vi "Unflatten (offset).vi"(8 "error in (no error)":errorcluster, 9 "offset (0)":i32, 10 "JSON stream":string, 11 "JSON Object In":refnum<class "JSON Object.lvclass">) -> (0 "error out":errorcluster, 1 "offset":i32, 3 "JSON Object Out":refnum<class "JSON Object.lvclass">, 4 "Empty?":bool)   [LabVIEW 2011, in "JSON Object.lvclass"]
uses:
  JSON Object.lvclass
  JSON Value/JSON Value.lvclass
  JSON Object.lvclass/JSON Object.ctl
  JSON Scalar/Strip Quotes.vi
  JSON Scalar/Parse In String (offset).vi
  JSON Scalar/Unescape JSON string.vi
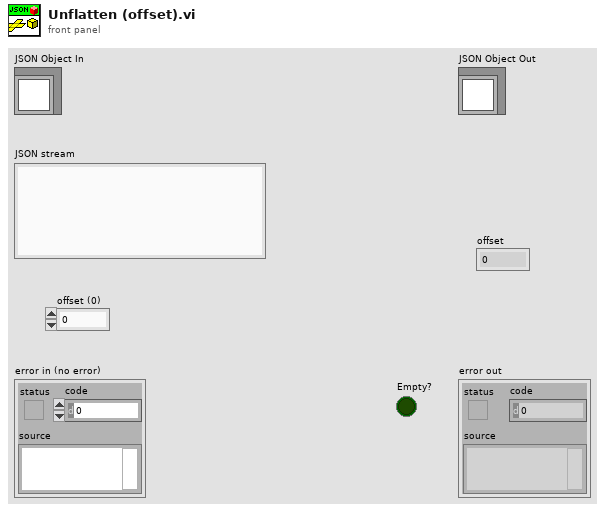
[diagram p1: front panel]
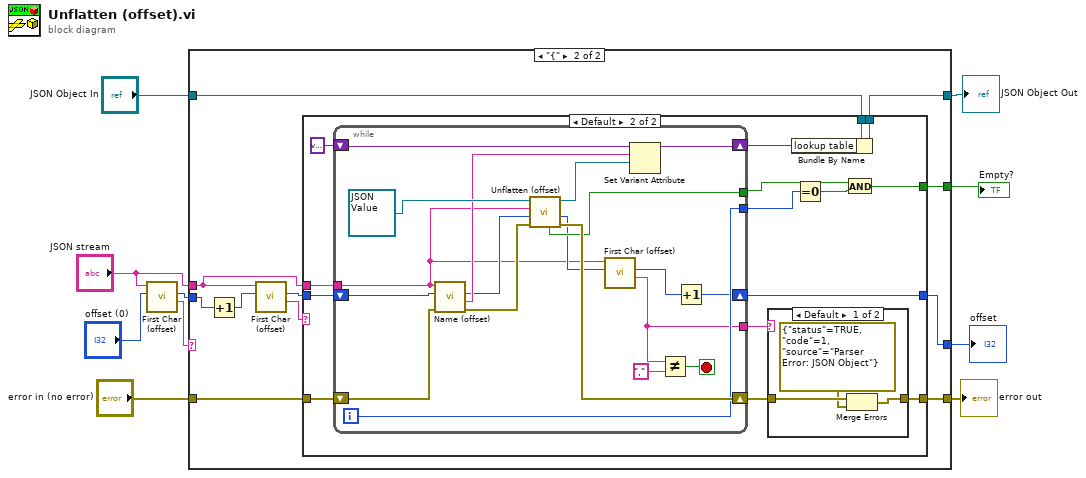
[diagram p0: block diagram]
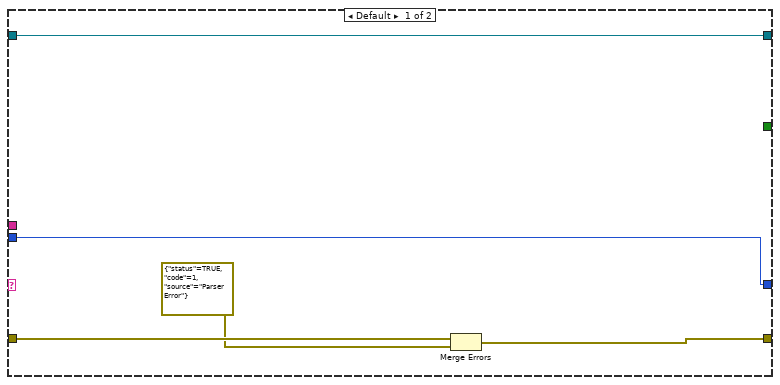
[diagram p2: hidden frame]
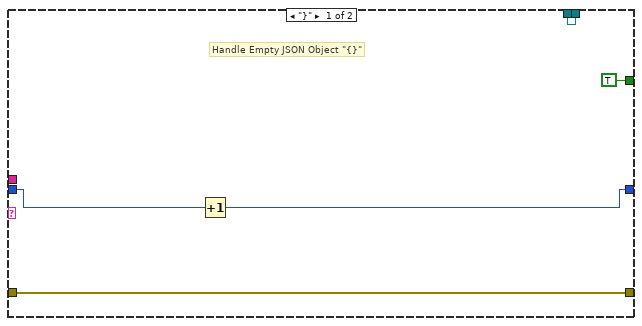
[diagram p3: hidden frame]
diagram:
  n1 = call "First Char (offset).vi"("offset (0)"="offset (0)", "String in"="JSON stream") -> ("First Char"=w10:string, "Offset"=w3:i32)  [unwired: 8 in]
  n2 = case shown="\"{\"" w10 {
    tunnel: "JSON stream" -> [_ w16]
    tunnel: [w15 w23] -> w9
    tunnel: "error in (no error)" -> [w12 w24]
    tunnel: [w14 w25] -> w7
    tunnel: "JSON Object In" -> [w14 w26]
    tunnel: [_ w22] -> w5
    tunnel: w3 -> [w13 w20]
    tunnel: [w13 w17] -> w2
    frame Default {
      n3 = Merge Errors(w12, errorcluster {"status"=TRUE, "code"=1, "source"="Parser Error"} ("error in")) -> (w15:errorcluster)
    }
    frame "{" {
      n4 = Increment(x=w20) -> (x+1=w19:i32)
      n5 = call "First Char (offset).vi"("offset (0)"=w19, "String in"=w16) -> ("First Char"=w21:string, "Offset"=w18:i32)  [unwired: 8 in]
      n6 = case shown="Default" w21 {
        tunnel: w16 -> [_ w46]
        tunnel: w26 -> [w31 w45]
        tunnel: [w31 w44] -> w25
        tunnel: w24 -> [w29 w43]
        tunnel: [w29 w41] -> w23
        tunnel: [TRUE w34] -> w22
        tunnel: w18 -> [w28 w33]
        tunnel: [w27 w32] -> w17
        frame "}" {
          # "Handle Empty JSON Object \"{}\""
          n7 = Increment(x=w28) -> (x+1=w27:i32)
        }
        frame Default {
          n8 = while {
            tunnel: [w58] -> w42
            shift-right: [w67] -> w40
            shift-left: w43 -> [w60]
            shift-right: [w63] -> w38
            shift-left: variant -> [w62]
            tunnel: [w55] -> w36
            tunnel: [w61] -> w37
            shift-right: [w53] -> w32
            shift-left: w33 -> [w57]
            tunnel: w46 -> [w51]
            i -> [w61]
            stop <- w68 stop-if-true
            n9 = call "Name (offset).vi"("error in (no error)"=w60, "offset (0)"=w57, "JSON"=w51) -> ("error out"=w59:errorcluster, "JSON name"=w65:string, "offset"=w56:i32)  [unwired: 6 in]
            n10 = call-dynamic "Unflatten (offset).vi"("error in (no error)"=w59, "offset (0)"=w56, "JSON stream"=w51, "JSON Value in"=refnum<class "JSON Value.lvclass"> refnum ("JSON Value.lvclass")) -> ("error out"=w67:errorcluster, "offset"=w54:i32, "JSON Value out"=w64:refnum<class "JSON Value.lvclass">, "Empty?"=w55:bool)  [unwired: 4 in]
            n11 = call "First Char (offset).vi"("offset (0)"=w54, "String in"=w51) -> ("First Char"=w58:string, "Offset"=w52:i32)  [unwired: 8 in]
            n12 = Set Variant Attribute(Variant=w62, name=w65, value=w64) -> (Variant out=w63:variant)  [unwired: 1 in, 2 out]
            n13 = Not Equal?(x=w58, y=",") -> (x != y?=w68:bool)
            n14 = Increment(x=w52) -> (x+1=w53:i32)
          }
          n15 = case shown="Default" w42 {
            tunnel: [w49 w50] -> w41
            tunnel: w40 -> [w48 w50]
            frame Default {
              n16 = Merge Errors(w48, errorcluster {"status"=TRUE, "code"=1, "source"="Parser Error: JSON Object"} ("error in")) -> (w49:errorcluster)
            }
            frame "}" {
            }
          }
          n17 = Bundle By Name(cluster=w45, "lookup table"=w38) -> (w44:refnum<class "JSON Object.lvclass">)
          n18 = Equal To 0?(x=w37) -> (x = 0?=w35:bool)
          n19 = And(x=w36, y=w35) -> (x .and. y?=w34:bool)
        }
      }
    }
  }
  "error out" <- w9
  "JSON Object Out" <- w7
  "Empty?" <- w5
  "offset" <- w2
